vi "Show Open VIs.vi"(6 "Variant in":variant, 7 "Shift Pressed?":bool, 8 "error in (no error)":errorcluster, 10 "QD Combo Box Ref":refnum<vi>, 11 "QD Launch VI Ref":refnum<vi>) -> (0 "error out":errorcluster, 4 "Variant out":variant)   [LabVIEW 2011]
doc: "Shows the VIs that are currently open. This brings up a dialog with the icons shown in a window that scales properly, and allow to open front panels, block diagrams, abort VIs, and show explorer window to the VI on disk. Add the Shift modifier to this quick drop function to open an explorer window to the VI.\n\nDefault Shortcut - [7]"
uses:
  <vilib>/Utility/traverseref.llb/TRef TravTarget.ctl
  <userlib>/_OpenG.lib/error/error.llb/Build Error Cluster__ogtk.vi
  <userlib>/_OpenG.lib/file/file.llb/Strip Path - Traditional__ogtk.vi
  <vilib>/Utility/traverseref.llb/VI Scripting - Traverse.lvlib
panel:
  in  "Undo Name":string="Quick Drop Keyboard Shortcut"
  # "Do not change the connector pane of this VI.\n\nSee the block diagram for directions on how to use this template."
  # "Specify the name of the Undo transaction"
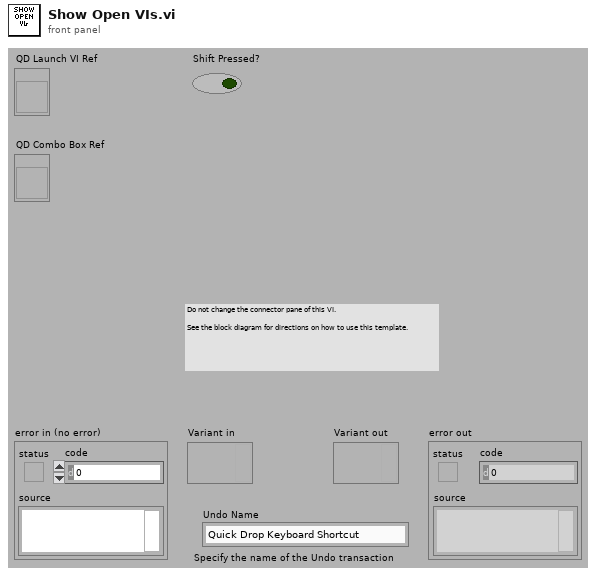
[diagram p1: front panel]
types:
  T1 = typedef "TRef TravTarget.ctl" = enum16{"FP", "BD", "Other"}
  T2 = typedef "LVRectTypeDef.ctl" = cluster{"left":i16, "top":i16, "right":i16, "bottom":i16}
  T3 = enum32{"Bad", "Idle", "Run top level", "Running"}
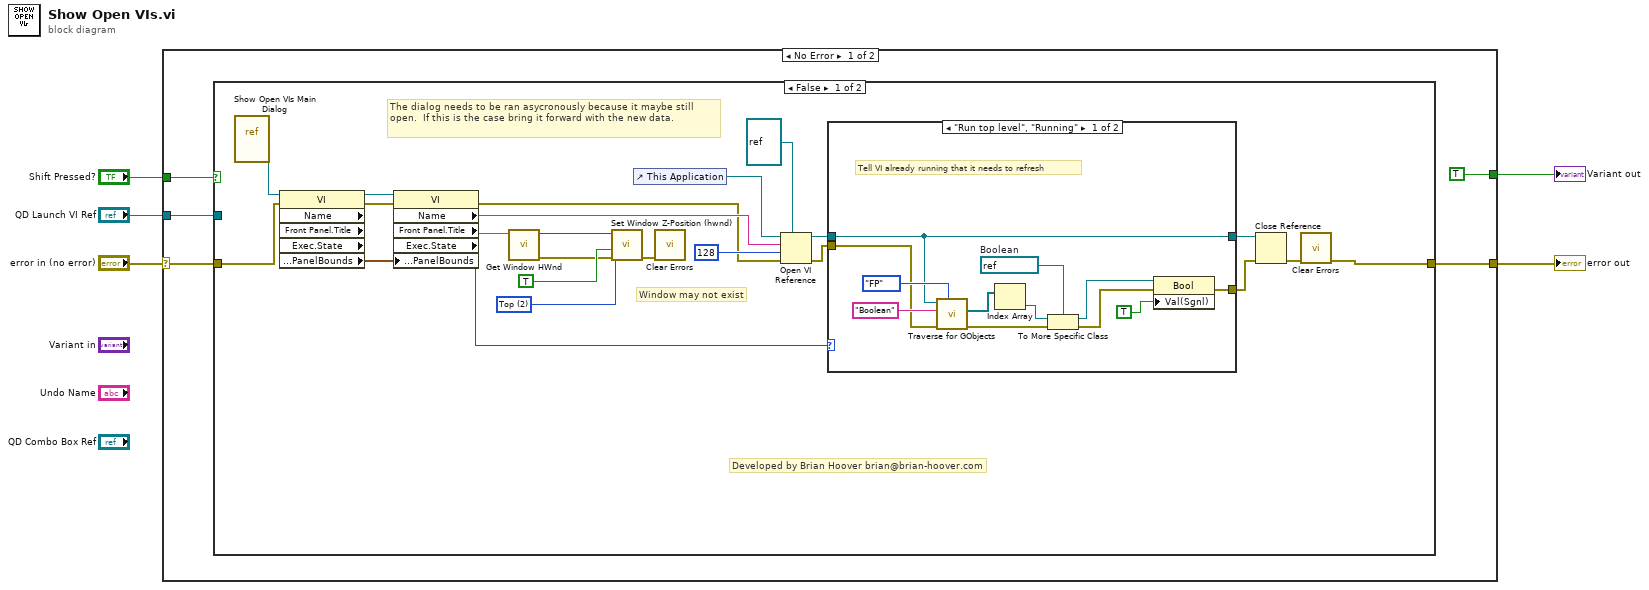
[diagram p0: block diagram]
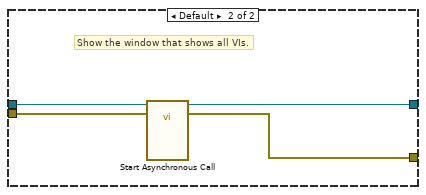
[diagram p2: hidden frame]
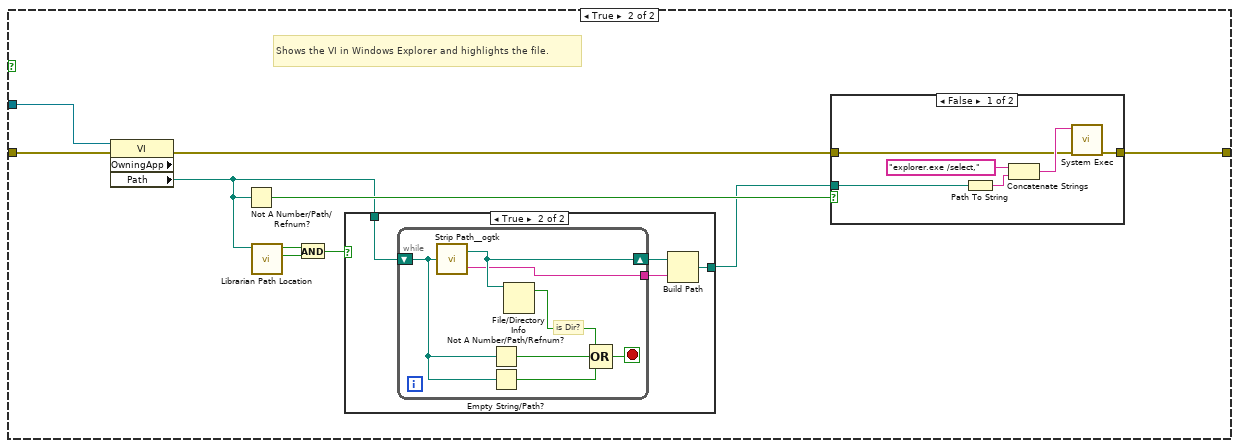
[diagram p3: hidden frame]
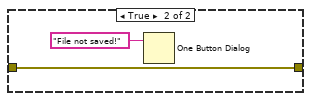
[diagram p5: hidden frame]
diagram:
  n1 = case shown="No Error" "error in (no error)" {
    selector: "error in (no error)" -> [w9 w80]
    tunnel: [w8 w80] -> w5
    tunnel: "QD Launch VI Ref" -> [w10 _]
    tunnel: [TRUE _] -> w4
    tunnel: "Shift Pressed?" -> [w7 _]
    frame No Error {
      n2 = case shown="False" w7 {
        tunnel: w10 -> [_ w59]
        tunnel: w9 -> [w13 w58]
        tunnel: [w16 w57] -> w8
        frame False {
          w19 = i16 2 items=["Not Topmost", "Topmost", "Top", "Bottom"] ("Z-Order Position")
          # "Developed by Brian Hoover brian@brian-hoover.com"
          # "The dialog needs to be ran asycronously because it maybe still open.  If this is the case bring it forward with the new data."
          # "Window may not exist"
          n3 = vi-ref "Show Open VIs Main Dialog.vi"() -> (w15:refnum<vi>)
          n4 = property class="VI" props=["Name", "Front Panel.Title", "Exec.State", "Front Panel.PanelBounds"](reference=w15, error in=w13) -> (reference out=w14:refnum<vi>, error out=w12:errorcluster, "Front Panel.PanelBounds"=w11:T2)  [unwired: 3 out]
          n5 = property class="VI"(reference=w14, error in=w12, "Front Panel.PanelBounds"=w11) -> (error out=w22:errorcluster, "Name"=w23:string, "Front Panel.Title"=w21:string, "Exec.State"=w32:T3)  [unwired: 1 out]
          n6 = call "Get Window HWnd.vi"("Window Name"=w21) -> ("error out"=w17:errorcluster, "HWnd Out"=w20:u32)  [unwired: 9 in]
          n7 = call "Set Window Z-Position (hwnd).vi"("error in (no error)"=w17, "Activate? (F)"=TRUE, "Z-Order Position"=w19, "HWnd"=w20) -> ("error out"=w25:errorcluster)  [unwired: 6 in, 1 out]
          n8 = control-ref of="This Application"() -> (w26:refnum<vi>)
          n9 = call <vilib>:"Clear Errors.vi"("error in (no error)"=w25) -> ()  [unwired: 6 in, 1 out]
          n10 = Open VI Reference(type specifier VI Refnum (for type only)=refnum<vi> refnum, application reference (local)=w26, vi path=w23, options=128, error in (no error)=w22) -> (vi reference=w28:refnum<vi>, error out=w31:errorcluster)  [unwired: 1 in]
          n11 = case shown="\"Run top level\", \"Running\"" w32 {
            tunnel: w28 -> [w35 w49]
            tunnel: [w35 w48] -> w30
            tunnel: w31 -> [w34 w47]
            tunnel: [w36 w46] -> w33
            frame "Run top level", "Running" {
              w41 = refnum<vi> refnum  # Boolean
              # "Tell VI already running that it needs to refresh"
              n12 = call <vilib>:"Traverse for GObjects.vi"("Traverse Target"=TRef_TravTarget."FP", "error in (no error)"=w34, "Class Name"="Boolean", "VI Refnum"=w35) -> ("error out"=w40:errorcluster, "References"=w43:refnum<vi>[])  [unwired: 4 in, 2 out]
              n13 = Index Array(array=w43) -> (element=w42:refnum<vi>)  [unwired: 1 in]
              n14 = To More Specific Class(target class=w41, reference=w42, error in=w40) -> (specific class reference=w38:refnum<vi>, error out=w37:errorcluster)
              n15 = property class="Bool"(reference=w38, error in=w37, "Val(Sgnl)"=TRUE) -> (error out=w36:errorcluster)  [unwired: 1 out]
            }
            frame Default {
              # "Show the window that shows all VIs."
              n16 = call-by-ref "Start Asynchronous Call"(reference=w49, error in=w47) -> (reference out=w48:refnum<vi>, error out=w46:errorcluster)  [unwired: 11 in, 1 out]
            }
          }
          n17 = Close Reference(reference=w30, error in (no error)=w33) -> (error out=w29:errorcluster)
          n18 = call <vilib>:"Clear Errors.vi"("error in (no error)"=w29) -> ("error out"=w16:errorcluster)  [unwired: 6 in]
        }
        frame True {
          # "Shows the VI in Windows Explorer and highlights the file."
          n19 = property class="VI" props=["OwningApp", "Path"](reference=w59, error in=w58) -> (error out=w55:errorcluster, "Path"=w51:path)  [unwired: 2 out]
          n20 = Not A Number/Path/Refnum?(number/path/refnum=w51) -> (NaN/Path/Refnum?=w56:bool)
          n21 = call <vilib>:"Librarian Path Location.vi"("path"=w51) -> ("path is to a file"=w53:bool, "path is in a VI library"=w54:bool)  [unwired: 6 in, 3 out]
          n22 = And(x=w54, y=w53) -> (x .and. y?=w52:bool)
          n23 = case shown="True" w52 {
            tunnel: w51 -> [w60 w64]
            tunnel: [w60 w61] -> w50
            frame False {
            }
            frame True {
              n24 = while {
                shift-right: [w66] -> w63
                shift-left: w64 -> [w68]
                tunnel: [w65] -> w62
                stop <- w70 stop-if-true
                # "is Dir?"
                n25 = call-poly <userlib>:"Strip Path__ogtk.vi"("path"=w68) -> ("stripped path"=w66:path, "name"=w65:string)
                n26 = Not A Number/Path/Refnum?(number/path/refnum=w68) -> (NaN/Path/Refnum?=w69:bool)
                n27 = Empty String/Path?(string/path=w68) -> (empty?=w67:bool)
                n28 = File/Directory Info(path=w66) -> (directory=w71:bool)  [unwired: 1 in, 6 out]
                n29 = Compound Arithmetic op=OR(w71, w69, w67) -> (w70:bool)
              }
              n30 = Build Path(base path=w63, name or relative path=w62) -> (appended path=w61:path)
            }
          }
          n31 = case shown="False" w56 {
            tunnel: [w74 w79] -> w57
            tunnel: w55 -> [w73 w79]
            tunnel: w50 -> [w72 _]
            frame False {
              n32 = Path To String(path=w72) -> (string=w76:string)
              n33 = Concatenate Strings("explorer.exe /select,", w76) -> (w75:string)
              n34 = call <vilib>:"System Exec.vi"("error in (no error)"=w73, "command line"=w75) -> ("error out"=w74:errorcluster)  [unwired: 6 in, 3 out]
            }
            frame True {
              n35 = One Button Dialog(message="File not saved!") -> ()  [unwired: 1 in, 1 out]
            }
          }
        }
      }
    }
    frame Error {
    }
  }
  "error out" <- w5
  "Variant out" <- w4
